vi "Get Clone Name.vi"() -> (1 "Clone ID":string, 2 "Clone Type":string)   [LabVIEW 2020, in "Actor Framework.lvlib"]
uses:
  Actor Framework.lvlib
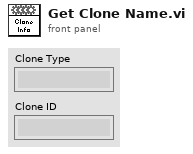
[diagram p1: front panel]
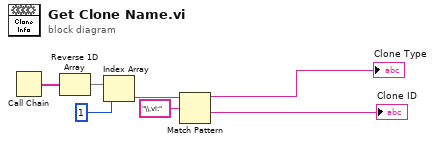
[diagram p0: block diagram]
diagram:
  n1 = Call Chain() -> (call chain=w3:string[])
  n2 = Reverse 1D Array(array=w3) -> (reversed array=w4:string[])
  n3 = Index Array(array=w4, index=1) -> (element=w5:string)
  n4 = Match Pattern(string=w5, regular expression="\\.vi:") -> (before substring=→"Clone Type":string, after substring=→"Clone ID":string)  [unwired: 1 in, 2 out]
